vi "ctrlManualThrusters.vi"() -> (10 "stop":bool, 14 "u_t0":dbl, 15 "u_t1":dbl, 16 "u_t2":dbl, 17 "alpha_t0":dbl, 18 "alpha_t1":dbl, 19 "alpha_t2":dbl)   [LabVIEW 2014]
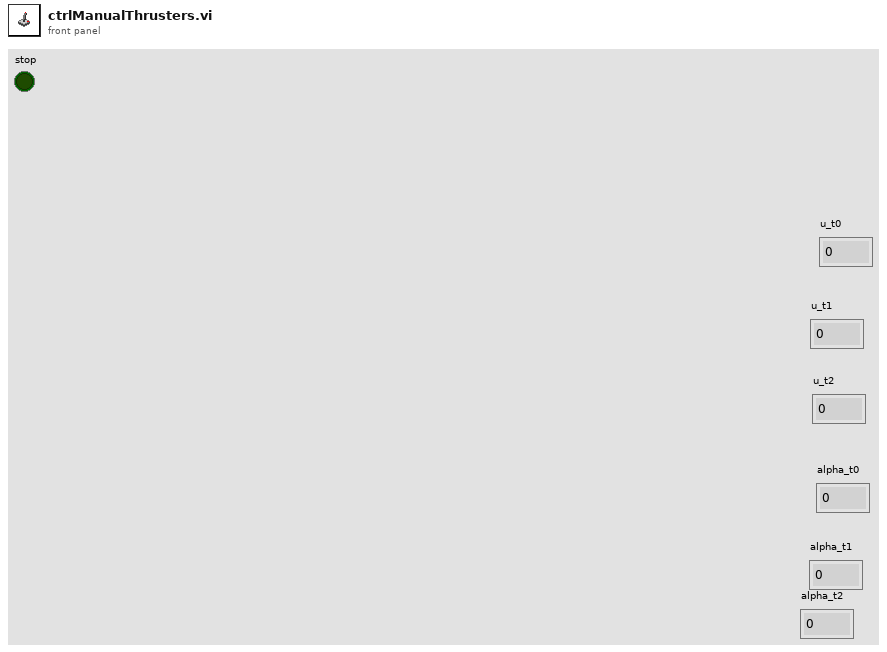
[diagram p1: front panel]
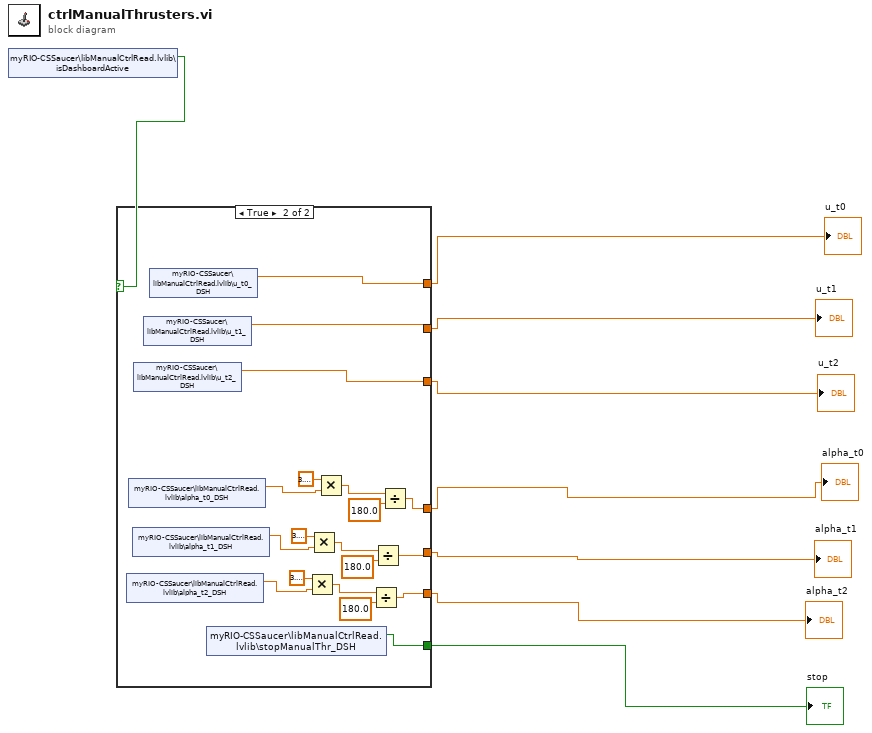
[diagram p0: block diagram]
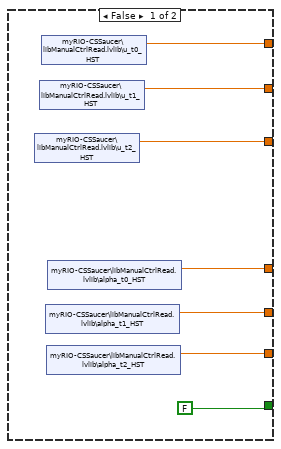
[diagram p2: hidden frame]
diagram:
  n1 = shared-variable "myRIO-CSSaucer\\libManualCtrlRead.lvlib\\isDashboardActive"() -> (w8:bool)  [unwired: 1 in, 1 out]
  n2 = case shown="True" w8 {
    tunnel: [w15 w34] -> w7
    tunnel: [w14 w33] -> w6
    tunnel: [w13 w32] -> w5
    tunnel: [w12 w18] -> w4
    tunnel: [w11 w17] -> w3
    tunnel: [w10 w16] -> w2
    tunnel: [FALSE w31] -> w1
    frame False {
      n3 = shared-variable "myRIO-CSSaucer\\libManualCtrlRead.lvlib\\u_t2_HST"() -> (w13:dbl)  [unwired: 1 in, 1 out]
      n4 = shared-variable "myRIO-CSSaucer\\libManualCtrlRead.lvlib\\u_t1_HST"() -> (w14:dbl)  [unwired: 1 in, 1 out]
      n5 = shared-variable "myRIO-CSSaucer\\libManualCtrlRead.lvlib\\u_t0_HST"() -> (w15:dbl)  [unwired: 1 in, 1 out]
      n6 = shared-variable "myRIO-CSSaucer\\libManualCtrlRead.lvlib\\alpha_t1_HST"() -> (w11:dbl)  [unwired: 1 in, 1 out]
      n7 = shared-variable "myRIO-CSSaucer\\libManualCtrlRead.lvlib\\alpha_t2_HST"() -> (w10:dbl)  [unwired: 1 in, 1 out]
      n8 = shared-variable "myRIO-CSSaucer\\libManualCtrlRead.lvlib\\alpha_t0_HST"() -> (w12:dbl)  [unwired: 1 in, 1 out]
    }
    frame True {
      n9 = shared-variable "myRIO-CSSaucer\\libManualCtrlRead.lvlib\\alpha_t2_DSH"() -> (w21:dbl)  [unwired: 1 in, 1 out]
      n10 = shared-variable "myRIO-CSSaucer\\libManualCtrlRead.lvlib\\alpha_t0_DSH"() -> (w19:dbl)  [unwired: 1 in, 1 out]
      n11 = shared-variable "myRIO-CSSaucer\\libManualCtrlRead.lvlib\\alpha_t1_DSH"() -> (w20:dbl)  [unwired: 1 in, 1 out]
      n12 = shared-variable "myRIO-CSSaucer\\libManualCtrlRead.lvlib\\u_t2_DSH"() -> (w32:dbl)  [unwired: 1 in, 1 out]
      n13 = shared-variable "myRIO-CSSaucer\\libManualCtrlRead.lvlib\\u_t1_DSH"() -> (w33:dbl)  [unwired: 1 in, 1 out]
      n14 = shared-variable "myRIO-CSSaucer\\libManualCtrlRead.lvlib\\u_t0_DSH"() -> (w34:dbl)  [unwired: 1 in, 1 out]
      n15 = shared-variable "myRIO-CSSaucer\\libManualCtrlRead.lvlib\\stopManualThr_DSH"() -> (w31:bool)  [unwired: 1 in, 1 out]
      n16 = Multiply(x=3.141592653589793, y=w21) -> (x*y=w25:dbl)
      n17 = Multiply(x=3.141592653589793, y=w20) -> (x*y=w22:dbl)
      n18 = Multiply(x=3.141592653589793, y=w19) -> (x*y=w28:dbl)
      n19 = Divide(x=w25, y=180.0) -> (x/y=w16:dbl)
      n20 = Divide(x=w22, y=180.0) -> (x/y=w17:dbl)
      n21 = Divide(x=w28, y=180.0) -> (x/y=w18:dbl)
    }
  }
  "u_t0" <- w7
  "u_t1" <- w6
  "u_t2" <- w5
  "alpha_t0" <- w4
  "alpha_t1" <- w3
  "alpha_t2" <- w2
  "stop" <- w1
